vi "Data2RGB.vi"(9 "SizeY":i64, 10 "SizeX":i64, 11 "Data":string) -> (3 "RGBarray":u32[][](array[numeric]))   [LabVIEW 2014]
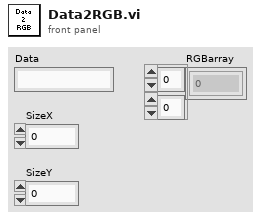
[diagram p1: front panel]
types:
  T1 = enum16{"big-endian, network order", "native, host order", "little-endian"}
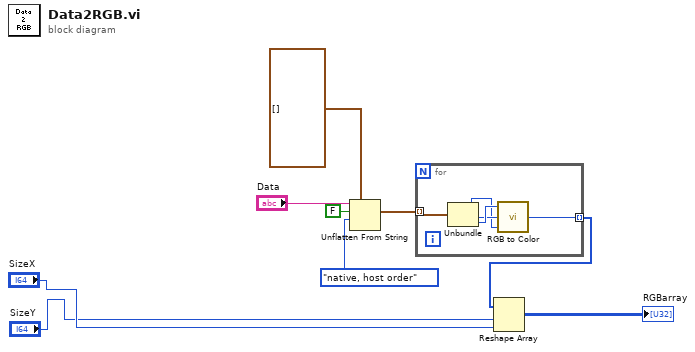
[diagram p0: block diagram]
diagram:
  n1 = Unflatten From String(type=cluster{"R":u8, "G":u8, "B":u8}[] [], binary string="Data", data includes array or string size? (T)=FALSE, byte order (0:big-endian, network order)=T1."native, host order") -> (value=w7:cluster{"R":u8, "G":u8, "B":u8}[])  [unwired: 1 in, 2 out]
  n2 = for {
    tunnel: w7 -> [w14] mode=indexing
    tunnel: [w13] -> w8 mode=indexing
    n3 = Unbundle(w14) -> ("R"=w10:u8, "G"=w11:u8, "B"=w12:u8)
    n4 = call <vilib>:"RGB to Color.vi"("B"=w10, "G"=w11, "R"=w12) -> ("Color"=w13:u32)
  }
  n5 = Reshape Array(w8, "SizeY", "SizeX") -> (→"RGBarray":u32[][])
